vi "Move Stage.vi"() -> ()   [LabVIEW 2016]
uses:
  C:/Program Files/Newport/Piezo Motion Control/Newport AG-UC2-UC8 Applet/Bin/AgilisCmdLib.DLL
  Program Files/Newport/Piezo Motion Control/Newport AG-UC2-UC8 Applet/Bin/AgilisCmdLib.DLL
panel:
  out "errstring 3":string
  out "errstring 2":string
  in  "stop":bool
  in  "Boolean":bool
  in  "NumberSteps":i64
  in  "controllerAddress":i32
  out "errstring":string
  out "error out":errorcluster={"status"=TRUE, "code"=1172, "source"="Invoke Node Error calling method Newport.AgilisCmdLib.AgilisCmds.ML, (System.ArgumentNullException: Key cannot be null.\r\nParameter name: key) <append><b>System.ArgumentNullException</b> in move_stage.vi"}
  out "ControllerVersion":string="AG-UC2 v2.2.0"
  out "VE":i32
  in  "Instrument Key":string="COM9"
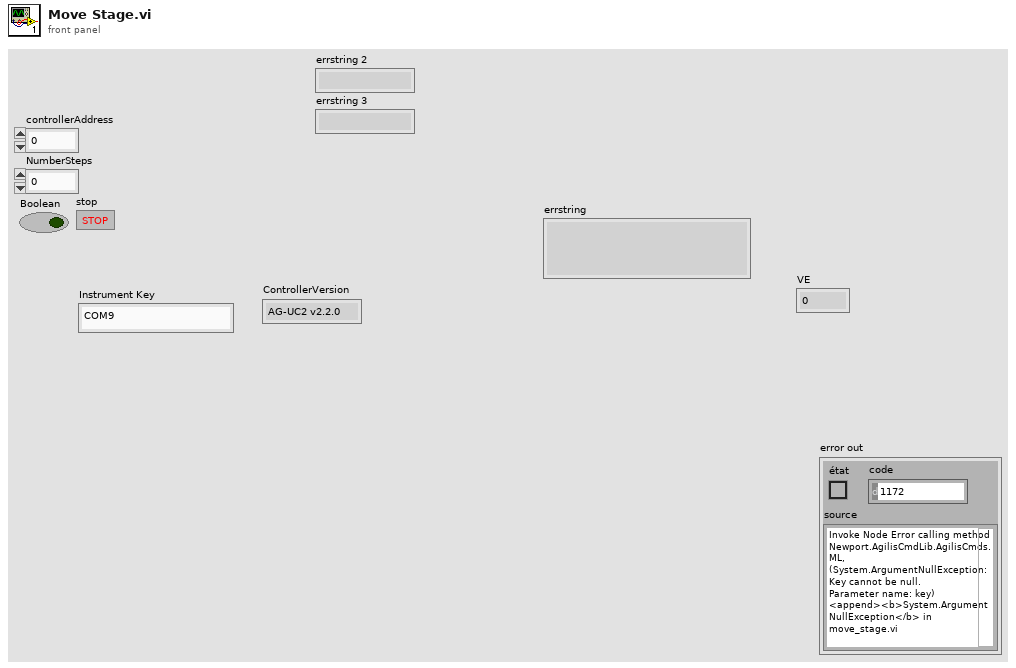
[diagram p1: front panel]
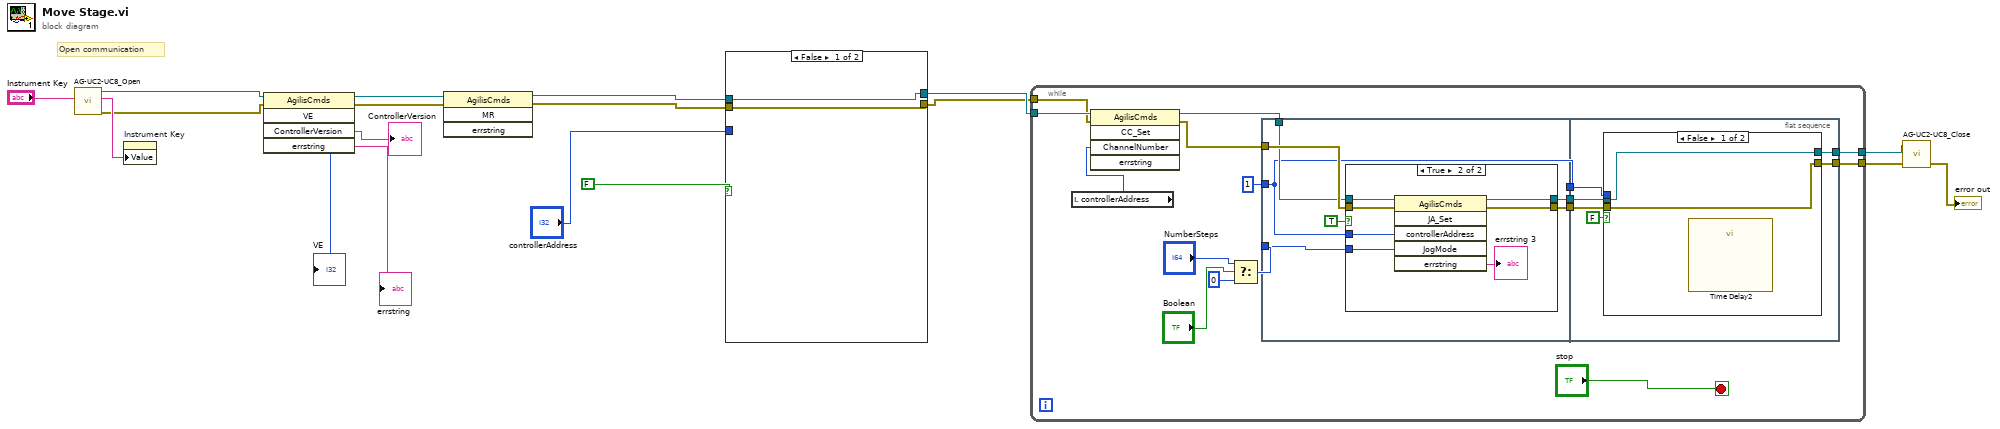
[diagram p0: block diagram]
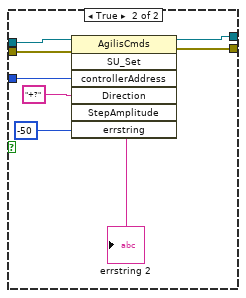
[diagram p2: hidden frame]
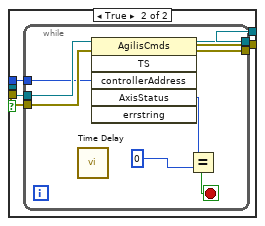
[diagram p4: hidden frame]
diagram:
  # "Open communication"
  n1 = call "AG-UC2-UC8_Open.vi"("Instrument Key IN"="Instrument Key") -> ("error out"=w16:errorcluster, "Instrument Key OUT"=w17:string, "AG-UC2-UC8 Reference"=w15:refnum<k24>)  [unwired: 3 in, 1 out]
  n2 = property on="Instrument Key" class="Str"("Value"=w17) -> ()  [unwired: 2 in, 2 out]
  n3 = invoke class="AgilisCmds" method="VE"(reference=w15, error in=w16) -> (reference out=w12:refnum<k24>, error out=w11:errorcluster, "VE"=→"VE":i32, "ControllerVersion"=→"ControllerVersion":string, "errstring"=→"errstring":string)  [unwired: 3 in]
  n4 = invoke class="AgilisCmds" method="MR"(reference=w12, error in=w11) -> (reference out=w6:refnum<k24>, error out=w5:errorcluster)  [unwired: 2 in, 2 out]
  n5 = case shown="False" FALSE {
    tunnel: w6 -> [w20 w28]
    tunnel: [w20 w27] -> w2
    tunnel: w5 -> [w19 w26]
    tunnel: [w19 w25] -> w1
    tunnel: "controllerAddress" -> [_ w22]
    frame False {
    }
    frame True {
      n6 = invoke class="AgilisCmds" method="SU_Set"(reference=w28, error in=w26, "controllerAddress"=w22, "Direction"="+?", "StepAmplitude"=-50) -> (reference out=w27:refnum<k24>, error out=w25:errorcluster, "errstring"=→"errstring 2":string)  [unwired: 2 in, 4 out]
    }
  }
  n7 = while {
    tunnel: [w41] -> w8
    tunnel: [w40] -> w7
    tunnel: w2 -> [w34]
    tunnel: w1 -> [w33]
    stop <- "stop" stop-if-true
    n8 = local read "controllerAddress"() -> (w30:i32)
    n9 = invoke class="AgilisCmds" method="CC_Set"(reference=w34, error in=w33, "ChannelNumber"=w30) -> (reference out=w32:refnum<k24>, error out=w31:errorcluster)  [unwired: 2 in, 3 out]
    n10 = Select(t="NumberSteps", s="Boolean", f=i64 0) -> (s? t:f=w35:i64)
    n11 = flat-sequence {
      tunnel: w31 -> [w51]
      tunnel: w32 -> [w50]
      tunnel: 1 ("controllerAddress") -> [w46]
      tunnel: w35 -> [w49]
      tunnel: [w48] -> w44
      tunnel: [w47] -> w43
      tunnel: [w46] -> w39
      tunnel: w44 -> [w66]
      tunnel: w43 -> [w65]
      tunnel: [w64] -> w41
      tunnel: [w63] -> w40
      tunnel: w39 -> [w62]
      frame #0 {
        n12 = case shown="True" TRUE {
          tunnel: w51 -> [w52 w60]
          tunnel: w50 -> [w53 w59]
          tunnel: w46 -> [_ w58]
          tunnel: w49 -> [_ w54]
          tunnel: [w53 w57] -> w48
          tunnel: [w52 w56] -> w47
          frame False {
          }
          frame True {
            n13 = invoke class="AgilisCmds" method="JA_Set"(reference=w59, error in=w60, "controllerAddress"=w58, "JogMode"=w54) -> (reference out=w57:refnum<k24>, error out=w56:errorcluster, "errstring"=→"errstring 3":string)  [unwired: 2 in, 3 out]
          }
        }
      }
      frame #1 {
        n14 = case shown="False" FALSE {
          tunnel: w66 -> [w68 w73]
          tunnel: w65 -> [w67 w72]
          tunnel: [w67 w71] -> w64
          tunnel: [w68 w70] -> w63
          tunnel: w62 -> [_ w69]
          frame False {
            n15 = call "Time Delay2"() -> ()  [unwired: 11 in, 1 out]
          }
          frame True {
            n16 = while {
              tunnel: w73 -> [w78]
              tunnel: w72 -> [w77]
              tunnel: [w76] -> w71
              tunnel: [w75] -> w70
              tunnel: w69 -> [w74]
              stop <- w81 stop-if-true
              n17 = call "Time Delay"() -> ()  [unwired: 11 in, 1 out]
              n18 = invoke class="AgilisCmds" method="TS"(reference=w78, error in=w77, "controllerAddress"=w74) -> (reference out=w75:refnum<k24>, error out=w76:errorcluster, "AxisStatus"=w80:i32)  [unwired: 3 in, 3 out]
              n19 = Equal?(x=w80, y=0) -> (x = y?=w81:bool)
            }
          }
        }
      }
    }
  }
  n20 = call "AG-UC2-UC8_Close.vi"("error in (no error)"=w8, "AG-UC2-UC8 Reference"=w7) -> ("Error out"=→"error out":errorcluster)  [unwired: 2 in, 1 out]
